vi "Is Runtime System.vi"(8 "错误输入（无错误）":errorcluster) -> (0 "错误输出":errorcluster, 3 "Is Runtime?":bool)   [LabVIEW 2012, in "Application.lvlib"]
uses:
  Application.lvlib
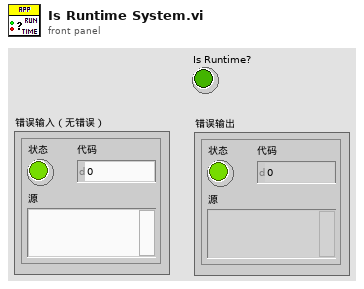
[diagram p1: front panel]
types:
  T1 = enum32{"invalid app kind", "Development System", "Run Time System", "Student Edition", "Embedded LabVIEW", "Evaluation", "Custom"}
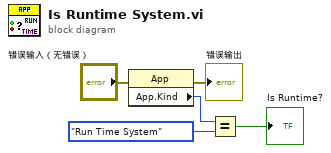
[diagram p0: block diagram]
diagram:
  n1 = property class="App"(error in="错误输入（无错误）") -> (error out=→"错误输出":errorcluster, "App.Kind"=w5:T1)  [unwired: 1 in, 1 out]
  n2 = Equal?(x=w5, y=T1."Run Time System" ("应用程序:类别")) -> (x = y?=→"Is Runtime?":bool)
